vi "MainMeasure.vi"(0 "TestSeqClass.lvclass":refnum<class "TestSeqClass.lvclass">, 5 "error in (no error)":errorcluster, 7 "Handles_In":T3={"MHM_Handle in"=0, "axis in"={"keyHandle"=0, "nodeId"=1}}) -> (13 "Handles_Out":T2, 14 "TestSeqClass out":refnum<class "TestSeqClass.lvclass">, 15 "TestMeasureStep out":refnum<class "TestMeasureStep.lvclass">, 19 "error out":errorcluster)   [LabVIEW 2019]
uses:
  TestMeasureStep/TestMeasureStep.lvclass
  testSeq/TestSeqClass.lvclass
  testSeq/TestSeqClass.lvclass/TestSeqClass.ctl
  GUIHandler_Main/GUI_Handler_Main.lvclass/GUI_Handler_Main.ctl
  ProgramSettings/ProgramSettings.lvclass/ProgramSettings.ctl
  testSeq/Typedef/TestStatus.ctl
  DUT_Interface/lv_interface/enums/MHM_WriteVerifyEnum.ctl
  DUT_Interface/lv_interface/enums/MHM_ParamEnum.ctl
  02676b47-250f-4f2d-8756-12bf81697de7.vi
  ProgramSettings/ProgramSettings.lvclass
  GUIHandler_Main/GUI_Handler_Main.lvclass
  DUT_Interface/lv_interface/MHM_1SL_interface.lvlib
  InstrumentsInterfaces/Motordriver/maxon EPOS/Examples/maxonEPOS.lvlib
  <instrlib>/Scancon ASIC/Scancon ASIC.lvlib
panel:
  in  "communication settings in":T1={"deviceName"="EPOS4", "protocolStackName"="MAXON SERIAL V2", "interfaceName"="USB", "portName"="USB0", "baudrate"=1000000, "timeout"=100}
  in  "UseCurrentTestPointer":bool=TRUE
  out "index":i32
  in  "Combo Box":string(combo)
  in  "nodeId":u32=1
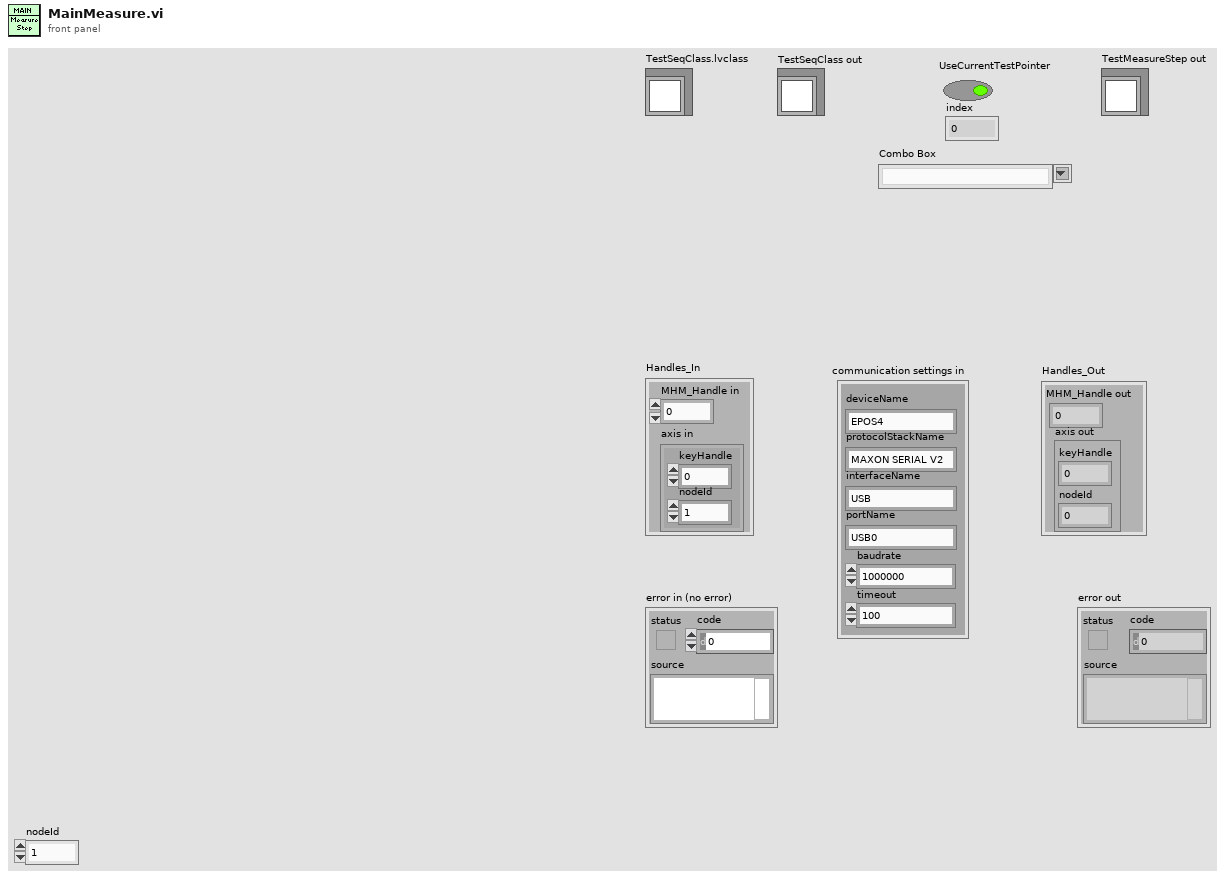
[diagram p1: front panel]
types:
  T1 = cluster{"deviceName":string, "protocolStackName":string, "interfaceName":string, "portName":string, "baudrate":u32, "timeout":u32}
  T2 = cluster{"MHM_Handle out":u32, "axis out":cluster{"keyHandle":u32, "nodeId":u16}}
  T3 = cluster{"MHM_Handle in":u32, "axis in":cluster{"keyHandle":u32, "nodeId":u16}}
  T4 = typedef "TestSeqType.ctl" = refnum<class "TestMeasureStep.lvclass">[]
  T5 = typedef "TestSeqClass.lvclass/TesstepType.ctl" = cluster{"TestName":string, "Meas":dbl, "Min ":dbl, "Max":dbl, "TestStatus":T6, "StringLimit":string, "StringMeas":string, "Unit":string}
  T6 = typedef "TestStatus.ctl" = enum16{"Not Executed", "Passed", "Failed", "Inconclusive", "Processing"}
  T7 = enum16{"MHM_NO_INTERFACE", "MHM_MB3U_SPI", "MHM_MB3U_BISS", "MHM_MB4U", "MHM_MB5U"}
  T8 = cluster{"profileAcceleration":u32, "profileDeceleration":u32}
  T9 = typedef "MHM_WriteVerifyEnum.ctl" = enum16{"MHM_SETONLY", "MHM_WRITE", "MHM_VERIFY"}
  T10 = typedef "MHM_ParamEnum.ctl" = enum16{"MHM_AVGFILT", "MHM_TLF", "MHM_DIR", "MHM_HYS", "MHM_RESO_MT", "MHM_RESO_ST", "MHM_CF_MTI", "MHM_SBL_MTI", "MHM_EBL_MTI", "MHM_GET_MTI", "MHM_CFG_IOP", "MHM_MT12", "MHM_RTX_MODE", "MHM_BIN_SSI", "MHM_EXT_SSI", "MHM_ENSSI", "MHM_VOSS", "MHM_VOSC", "MHM_CIBM", "MHM_ENF", "MHM_TEST", "MHM_GAINF", "MHM_GAINR", "MHM_GCC", "MHM_ENAC", "MHM_CRCS", "MHM_ENLC", "MHM_REGPROT", "MHM_INSPROT", "MHM_PRES_IO1", "MHM_DIR_IO2", "MHM_ENCMD3", "MHM_ENCMD2", "MHM_CRC_CFG", "MHM_OFFS_MT", "MHM_OFFS_ST", "MHM_CRC_OFFS", "MHM_PSET_MT", "MHM_PSET_ST", "MHM_CRC_PSET", "MHM_ERR_CFG", "MHM_ERR_OFFS", "MHM_ERR_POS", "MHM_ERR_EXT", "MHM_ERR_AMIN", "MHM_ERR_AMAX", "MHM_ERR_MTI", "MHM_ERR_MT", "MHM_GAIN", "MHM_EDSBANK", "MHM_PRO_ID", "MHM_DEV_ID0", "MHM_DEV_ID1", "MHM_DEV_ID2", "MHM_DEV_ID3", "MHM_DEV_ID4", "MHM_DEV_ID5", "MHM_MFG_ID0", "MHM_MFG_ID1", "MHM_HARMCAL", "MHM_DISBISS", "MHM_NTOA", "MHM_ENCMD01", "MHM_CHIP_REL"}
  T11 = cluster{"Konfigurations Filnavn":refnum<vi>, "Forsyningsspænding":refnum<vi>, "Kode":refnum<vi>, "Opløsning":refnum<vi>}
  T12 = typedef "ProgramSettings.lvclass/SettingParams.ctl" = cluster{"Serial Port for strømforsyning":refnum<visa-resource-name>, "Serial Port for SSI Interface":refnum<visa-resource-name>}
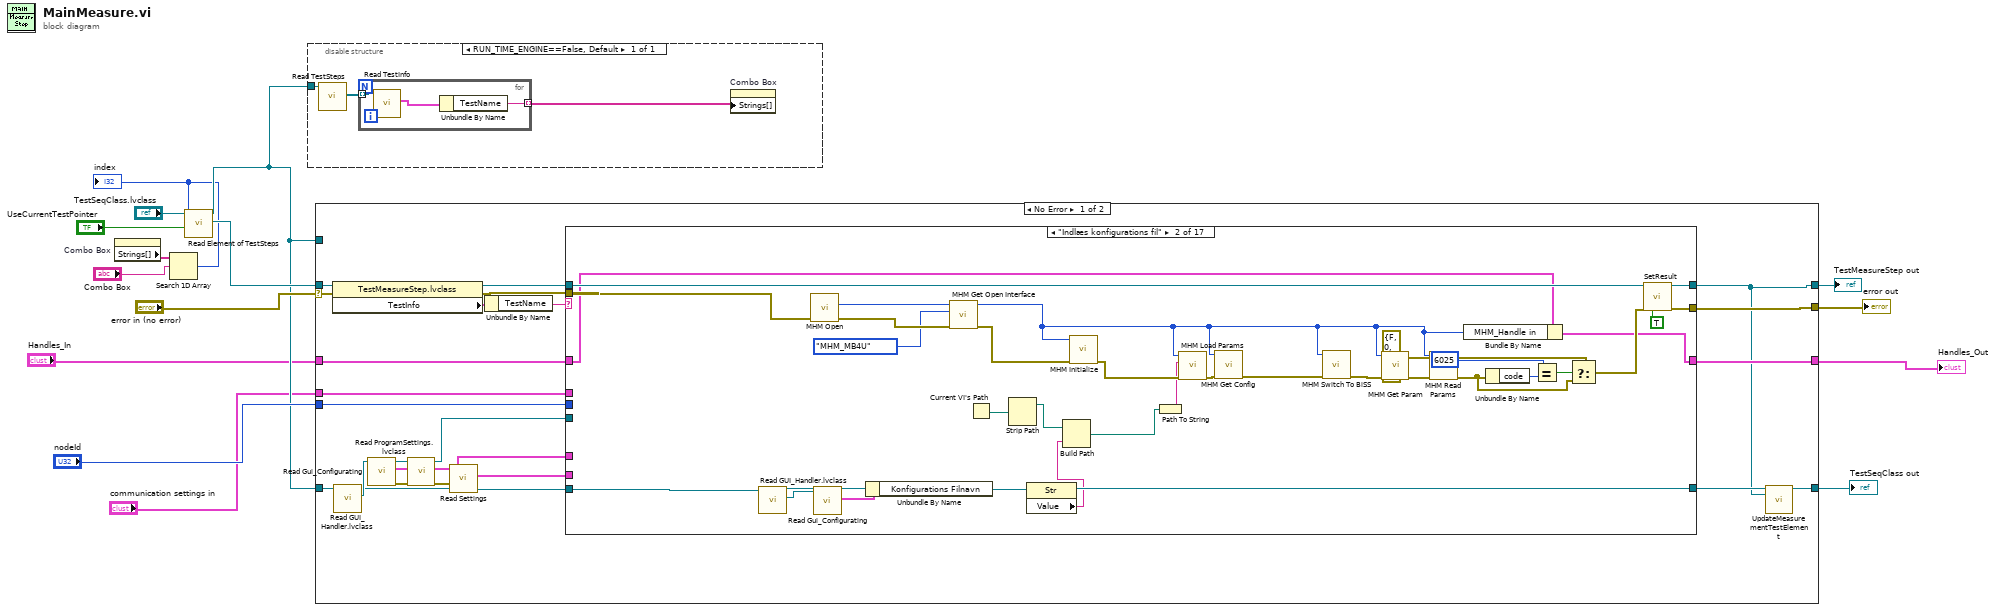
[diagram p0: block diagram]
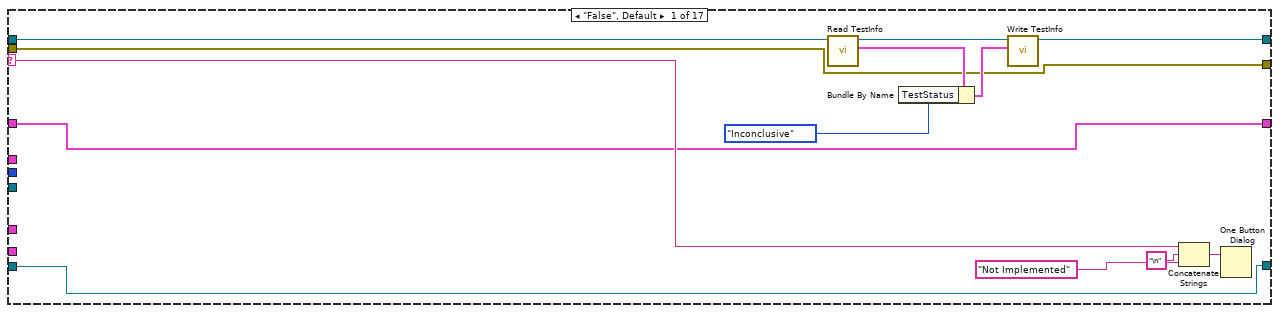
[diagram p2: hidden frame]
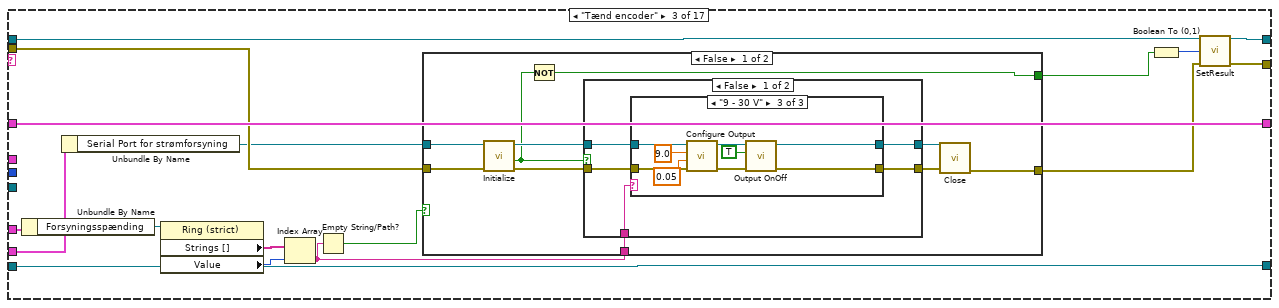
[diagram p3: hidden frame]
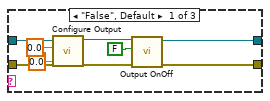
[diagram p4: hidden frame]
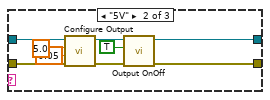
[diagram p5: hidden frame]
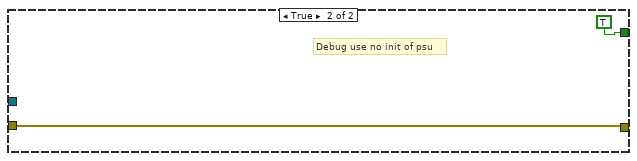
[diagram p7: hidden frame]
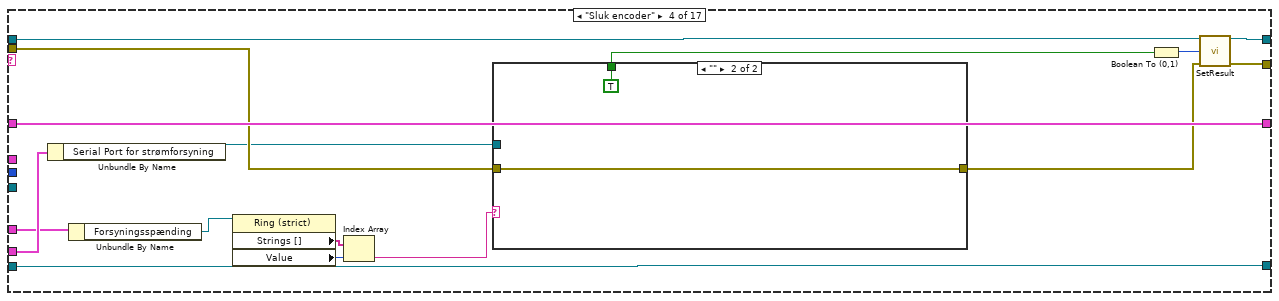
[diagram p8: hidden frame]
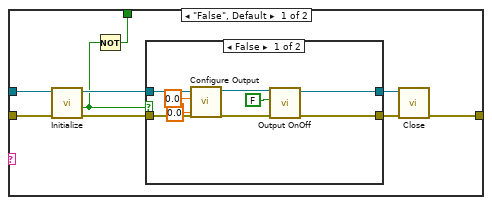
[diagram p9: hidden frame]
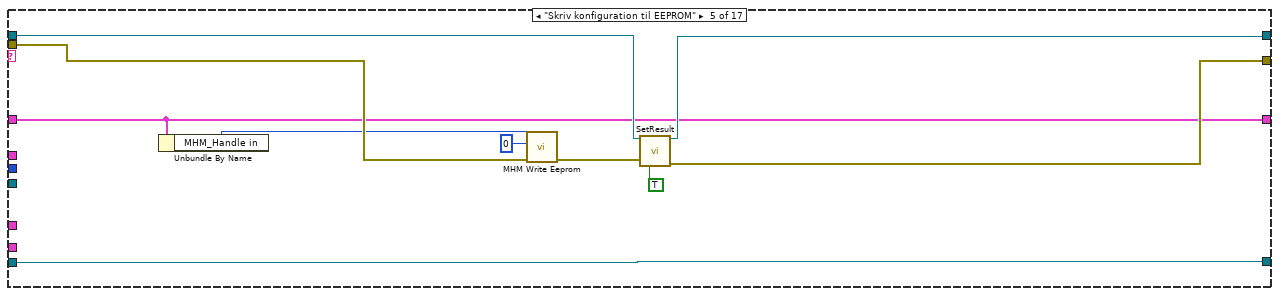
[diagram p11: hidden frame]
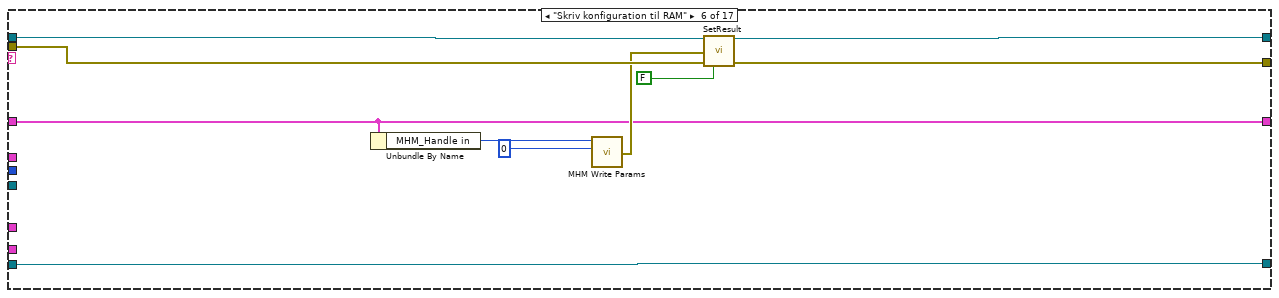
[diagram p12: hidden frame]
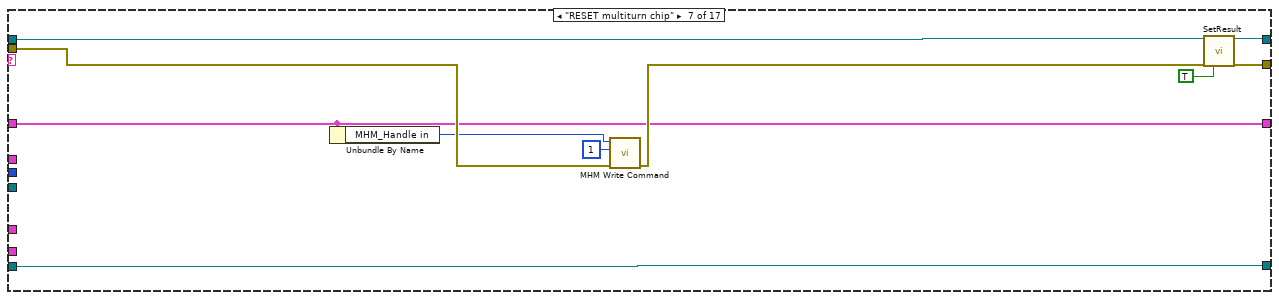
[diagram p13: hidden frame]
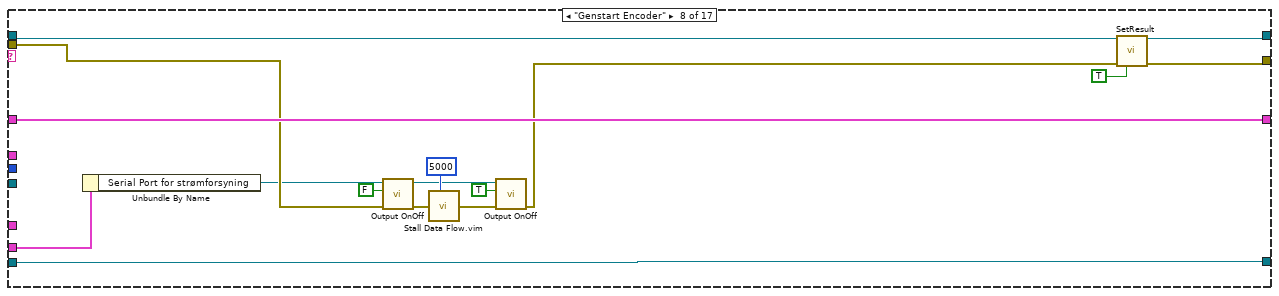
[diagram p14: hidden frame]
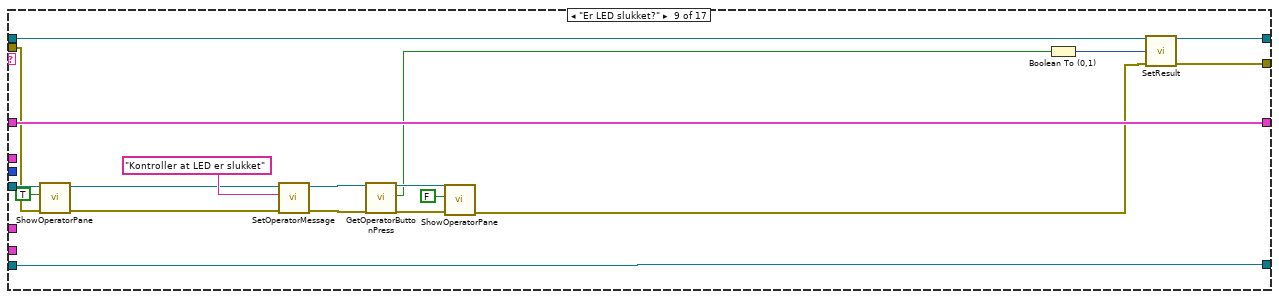
[diagram p15: hidden frame]
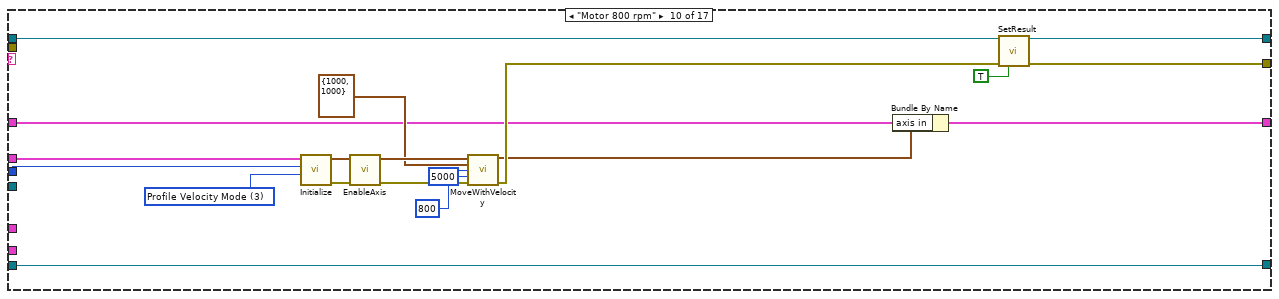
[diagram p16: hidden frame]
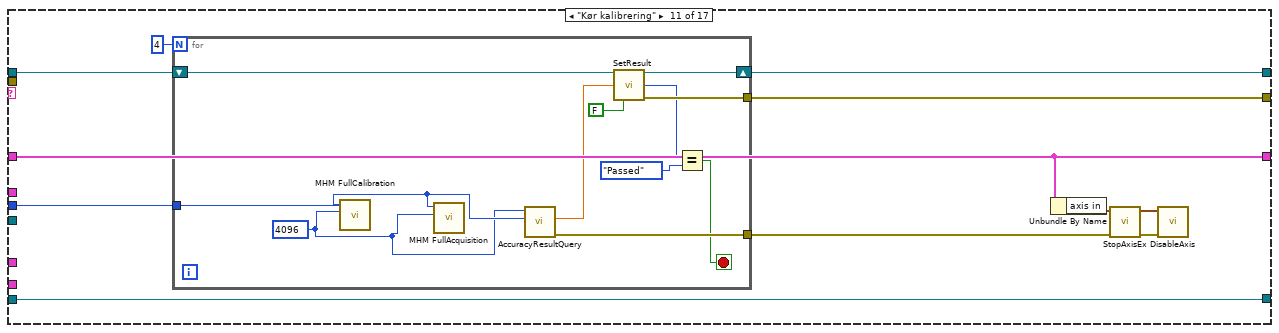
[diagram p17: hidden frame]
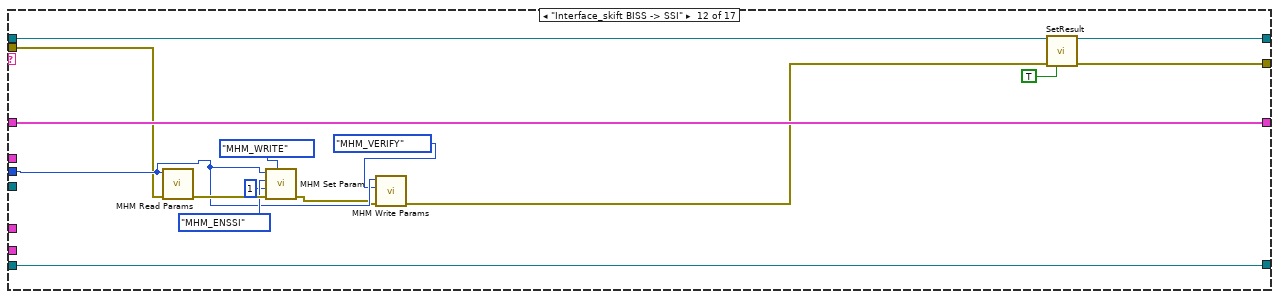
[diagram p18: hidden frame]
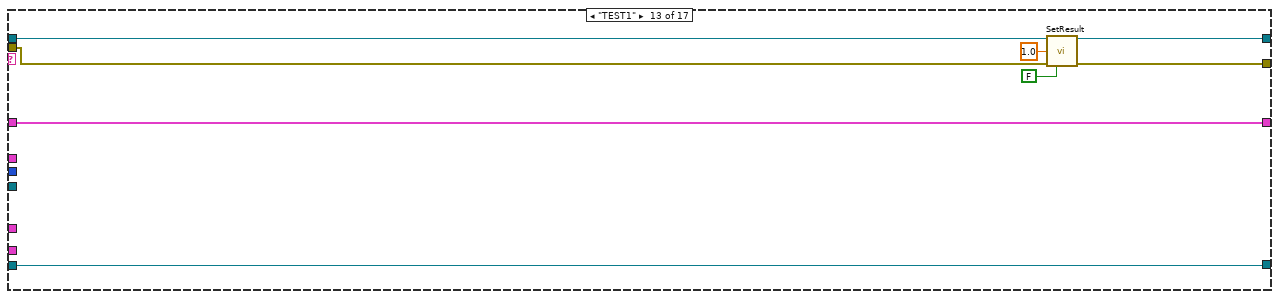
[diagram p19: hidden frame]
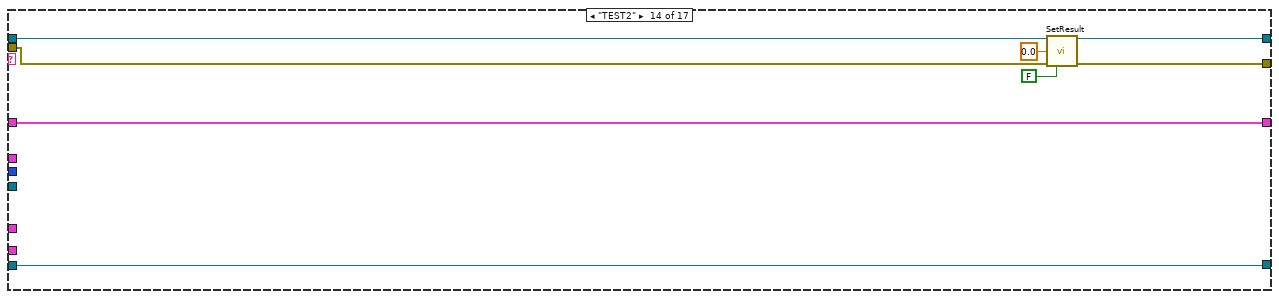
[diagram p20: hidden frame]
diagram:
  n1 = property on="Combo Box" class="CmbBox"() -> ("Strings[]"=w6:string[])  [unwired: 2 in, 2 out]
  n2 = Search 1D Array(1D array=w6, element="Combo Box") -> (index of element=w4:i32)  [unwired: 1 in]
  "index" <- w4
  n3 = call "Read Element of TestSteps.vi"("UseCurrentTestPointer"="UseCurrentTestPointer", "index"=w4, "TestSeqClass in"="TestSeqClass.lvclass") -> ("TestMeasureStep.lvclass"=w11:refnum<class "TestMeasureStep.lvclass">, "TestSeqClass out"=w8:refnum<class "TestSeqClass.lvclass">)  [unwired: 6 in, 1 out]
  n4 = disable-structure shown="RUN_TIME_ENGINE==False, Default" {
    disable-tunnel: w8 -> [w18]
    frame condition #0 (active) {
      n5 = call-dynamic "Read TestSteps.vi"("TestSeqClass in"=w18) -> ("TestSteps"=w17:T4)  [unwired: 8 in, 2 out]
      n6 = for {
        tunnel: w17 -> [w21] mode=indexing
        tunnel: [w19] -> w16 mode=indexing
        n7 = call-dynamic "Read TestInfo.vi"("TestMeasureStep in"=w21) -> ("TestInfo 2"=w20:T5)  [unwired: 8 in, 2 out]
        n8 = Unbundle By Name(w20) -> ("TestName"=w19:string)
      }
      n9 = property on="Combo Box" class="CmbBox"("Strings[]"=w16) -> ()  [unwired: 2 in, 2 out]
    }
  }
  n10 = case shown="No Error" "error in (no error)" {
    selector: "error in (no error)" -> [w38 w349]
    tunnel: [w36 w349] -> w14
    tunnel: [w33 w348] -> w13
    tunnel: w11 -> [w44 w348]
    tunnel: [w40 w347] -> w2
    tunnel: "Handles_In" -> [w39 w347]
    tunnel: w8 -> [w30 w346]
    tunnel: [w34 w346] -> w10
    tunnel: "nodeId" -> [w23 _]
    tunnel: w8 -> [_ _]
    tunnel: "communication settings in" -> [w22 _]
    frame No Error {
      n11 = property class="TestMeasureStep.lvclass"(reference=w44, error in=w38) -> (reference out=w42:refnum<class "TestMeasureStep.lvclass">, error out=w37:errorcluster, "TestInfo"=w43:T5)
      n12 = call-dynamic "Read GUI_Handler.lvclass.vi"("TestSeqClass in"=w30) -> ("GUI_Handler.lvclass"=w32:refnum<class "GUI_Handler_Main.lvclass">)  [unwired: 8 in, 2 out]
      n13 = call-dynamic "Read Gui_Configurating.vi"("GUI_Handler_Main in"=w32) -> ("error out"=w26:errorcluster, "Gui_Configurating"=w31:T11, "GUI_Handler_Main out"=w29:refnum<class "GUI_Handler_Main.lvclass">)  [unwired: 8 in]
      n14 = call "Read ProgramSettings.lvclass.vi"("error in (no error)"=w26, "GUI_Handler_Main in"=w29) -> ("error out"=w28:errorcluster, "ProgramSettings.lvclass"=w27:refnum<class "ProgramSettings.lvclass">, "GUI_Handler_Main out"=w24:refnum<class "GUI_Handler_Main.lvclass">)  [unwired: 7 in]
      n15 = call "Read Settings.vi"("error in (no error)"=w28, "ProgramSettings in"=w27) -> ("Settings"=w25:T12)  [unwired: 7 in, 2 out]
      n16 = Unbundle By Name(w43) -> ("TestName"=w41:string)
      n17 = case shown="\"Indlæs konfigurations fil\"" w41 {
        selector: w41 -> [w56 _ _ _ _ _ _ _ _ _ _ _ _ _ _ _ _]
        tunnel: w42 -> [w53 w90 w104 w165 w195 w204 w213 w221 w249 w260 w281 w304 w311 w319 w331 w336 w345]
        tunnel: [w48 w89 w103 w164 w192 w203 w212 w220 w248 w259 w280 w303 w310 w318 w331 w335 w345] -> w33
        tunnel: [w47 w60 w107 w168 w190 w200 w209 w233 w252 w254 w277 w308 w316 w324 w330 w341 w344] -> w40
        tunnel: w39 -> [w47 w59 w107 w168 w190 w200 w209 w233 w252 w255 w277 w308 w316 w324 w330 w341 w344]
        tunnel: w37 -> [w45 w88 w106 w167 w197 w207 w215 w231 w243 _ _ w295 w313 w321 w328 w332 w342]
        tunnel: w30 -> [w46 w87 w105 w166 w199 w208 w217 w232 w251 w271 w282 w307 w315 w323 w329 w340 w343]
        tunnel: [w46 w83 w105 w166 w199 w208 w217 w232 w251 w271 w282 w307 w315 w323 w329 w340 w343] -> w35
        tunnel: [w45 w82 w97 w159 w193 w207 w214 w219 w247 w258 w279 w306 w314 w322 w328 w334 w342] -> w36
        tunnel: w31 -> [_ _ w101 w157 _ _ _ _ _ _ _ _ _ _ _ _ _]
        tunnel: w25 -> [_ _ w100 w162 _ _ _ w230 _ _ _ _ _ _ w326 _ _]
        tunnel: w24 -> [_ _ _ _ _ _ _ _ w246 _ _ _ _ _ _ _ _]
        tunnel: w23 -> [_ _ _ _ _ _ _ _ _ w266 w278 w298 _ _ _ w339 _]
        tunnel: w22 -> [_ _ _ _ _ _ _ _ _ w253 _ _ _ _ _ _ _]
        frame "False", Default {
          n18 = call-dynamic "Read TestInfo.vi"("TestMeasureStep in"=w53) -> ("TestInfo 2"=w52:T5, "TestMeasureStep out"=w49:refnum<class "TestMeasureStep.lvclass">)  [unwired: 8 in, 1 out]
          n19 = Bundle By Name(cluster=w52, "TestStatus"=TestStatus."Inconclusive") -> (w50:T5)
          n20 = call-dynamic "Write TestInfo.vi"("TestInfo 2"=w50, "TestMeasureStep in"=w49) -> ("TestMeasureStep out"=w48:refnum<class "TestMeasureStep.lvclass">)  [unwired: 8 in, 1 out]
          n21 = Concatenate Strings(w56, "\n" ("string"), "Not Implemented" ("string")) -> (w57:string)
          n22 = One Button Dialog(message=w57) -> ()  [unwired: 1 in, 1 out]
        }
        frame "Indlæs konfigurations fil" {
          n23 = call-dynamic "Read GUI_Handler.lvclass.vi"("TestSeqClass in"=w87) -> ("GUI_Handler.lvclass"=w86:refnum<class "GUI_Handler_Main.lvclass">, "TestSeqClass out"=w83:refnum<class "TestSeqClass.lvclass">)  [unwired: 8 in, 1 out]
          n24 = call "MHM Open.vi"("error in (no error)"=w88) -> ("error out"=w65:errorcluster, "pulMHMHandle"=w62:u32)  [unwired: 8 in, 1 out]
          n25 = call-dynamic "Read Gui_Configurating.vi"("GUI_Handler_Main in"=w86) -> ("Gui_Configurating"=w85:T11)  [unwired: 8 in, 2 out]
          n26 = Unbundle By Name(w85) -> ("Konfigurations Filnavn"=w84:refnum<vi>)
          n27 = call "MHM Get Open Interface.vi"("error in (no error)"=w65, "ulInterface"=T7."MHM_MB4U" ("MHM_InterfaceEnum"), "ulMHMHandle"=w62) -> ("error out"=w64:errorcluster, "ulMHMHandle out"=w58:u32)  [unwired: 7 in]
          n28 = Current VI's Path() -> (path=w67:path)
          n29 = Strip Path(path=w67) -> (stripped path=w66:path)  [unwired: 1 out]
          n30 = property class="Str"(reference=w84) -> ("Value"=w69:string)  [unwired: 1 in, 2 out]
          n31 = Build Path(base path=w66, name or relative path=w69) -> (appended path=w68:path)
          n32 = call "MHM Initialize.vi"("error in (no error)"=w64, "ulMHMHandle"=w58) -> ("error out"=w81:errorcluster)  [unwired: 8 in, 1 out]
          n33 = Path To String(path=w68) -> (string=w70:string)
          n34 = call "MHM Load Params.vi"("error in (no error)"=w81, "pcFilename"=w70, "ulMHMHandle"=w58) -> ("error out"=w71:errorcluster)  [unwired: 7 in, 1 out]
          n35 = call "MHM Get Config.vi"("error in (no error)"=w71, "ulMHMHandle"=w58) -> ("error out"=w72:errorcluster)  [unwired: 7 in, 2 out]
          n36 = call "MHM Switch To BiSS.vi"("error in (no error)"=w72, "ulMHMHandle"=w58) -> ("error out"=w73:errorcluster)  [unwired: 7 in, 2 out]
          n37 = call "MHM Get Param.vi"("error in (no error)"=w73, "ulMHMHandle"=w58) -> ("error out"=w74:errorcluster)  [unwired: 7 in, 2 out]
          n38 = call "MHM Read Params.vi"("error in (no error)"=w74, "ulMHMHandle"=w58) -> ("error out"=w75:errorcluster)  [unwired: 8 in, 1 out]
          n39 = Bundle By Name(cluster=w59, "MHM_Handle in"=w58) -> (w60:T3)
          n40 = Unbundle By Name(w75) -> ("code"=w80:i32)
          n41 = Equal?(x=6025, y=w80) -> (x = y?=w78:bool)
          n42 = Select(t=errorcluster {"status"=FALSE, "code"=0, "source"=""}, s=w78, f=w75) -> (s? t:f=w76:errorcluster)
          n43 = call "SetResult.vi"("TestMeasureStep in"=w90, "error in (no error)"=w76, "Use Error As result"=TRUE) -> ("TestMeasureStep out"=w89:refnum<class "TestMeasureStep.lvclass">, "error out"=w82:errorcluster)  [unwired: 10 in, 1 out]
        }
        frame "Tænd encoder" {
          n44 = Unbundle By Name(w101) -> ("Forsyningsspænding"=w96:refnum<vi>)
          n45 = Unbundle By Name(w100) -> ("Serial Port for strømforsyning"=w99:refnum<visa-resource-name>)
          n46 = property class="Ring (strict)"(reference=w96) -> ("Strings []"=w95:string[], "Value"=w94:u16)  [unwired: 1 in, 2 out]
          n47 = Index Array(array=w95, index=w94) -> (element=w93:string)
          n48 = Empty String/Path?(string/path=w93) -> (empty?=w92:bool)
          n49 = case shown="False" w92 {
            tunnel: w106 -> [w117 w152]
            tunnel: w99 -> [w113 _]
            tunnel: [w112 w152] -> w98
            tunnel: w93 -> [w111 _]
            tunnel: [w108 TRUE ("Init failed")] -> w91
            frame False {
              n50 = call <instrlib>:"Initialize.vi"("error in (no error)"=w117, "VISA resource name"=w113) -> ("error out"=w110:errorcluster, "Init failed"=w109:bool, "VISA resource name out"=w116:refnum<visa-resource-name>)  [unwired: 6 in, 1 out]
              n51 = Not(x=w109) -> (.not. x?=w108:bool)
              n52 = case shown="False" w109 {
                tunnel: w116 -> [w122 w150]
                tunnel: w110 -> [w121 w149]
                tunnel: [w120 w150] -> w115
                tunnel: [w119 w149] -> w114
                tunnel: w111 -> [w118 _]
                frame False {
                  n53 = case shown="\"9 - 30 V\"" w118 {
                    tunnel: w122 -> [w126 w139 w148]
                    tunnel: w121 -> [w129 w133 w142]
                    tunnel: [w128 w136 w145] -> w120
                    tunnel: [w127 w132 w141] -> w119
                    frame "False", Default {
                      n54 = call <instrlib>:"Configure Output.vi"("Current Level (0.0 A)"=0.0, "Voltage Level (0.0 V)"=0.0, "VISA resource name"=w126) -> ("VISA resource name out"=w125:refnum<visa-resource-name>)  [unwired: 7 in, 1 out]
                      n55 = call <instrlib>:"Output OnOff.vi"("error in (no error)"=w129, "Output On/Off"=FALSE, "VISA resource name"=w125) -> ("error out"=w127:errorcluster, "VISA resource name out"=w128:refnum<visa-resource-name>)  [unwired: 7 in]
                    }
                    frame "5V" {
                      n56 = call <instrlib>:"Configure Output.vi"("error in (no error)"=w133, "Current Level (0.0 A)"=0.05, "Voltage Level (0.0 V)"=5.0, "VISA resource name"=w139) -> ("error out"=w135:errorcluster, "VISA resource name out"=w138:refnum<visa-resource-name>)  [unwired: 6 in]
                      n57 = call <instrlib>:"Output OnOff.vi"("error in (no error)"=w135, "Output On/Off"=TRUE, "VISA resource name"=w138) -> ("error out"=w132:errorcluster, "VISA resource name out"=w136:refnum<visa-resource-name>)  [unwired: 7 in]
                    }
                    frame "9 - 30 V" {
                      n58 = call <instrlib>:"Configure Output.vi"("error in (no error)"=w142, "Current Level (0.0 A)"=0.05, "Voltage Level (0.0 V)"=9.0, "VISA resource name"=w148) -> ("error out"=w144:errorcluster, "VISA resource name out"=w147:refnum<visa-resource-name>)  [unwired: 6 in]
                      n59 = call <instrlib>:"Output OnOff.vi"("error in (no error)"=w144, "Output On/Off"=TRUE, "VISA resource name"=w147) -> ("error out"=w141:errorcluster, "VISA resource name out"=w145:refnum<visa-resource-name>)  [unwired: 7 in]
                    }
                  }
                }
                frame True {
                }
              }
              n60 = call <instrlib>:"Close.vi"("error in (no error)"=w114, "VISA resource name"=w115) -> ("error out"=w112:errorcluster)  [unwired: 9 in]
            }
            frame True {
              # "Debug use no init of psu"
            }
          }
          n61 = Boolean To (0,1)(Boolean=w91) -> (0, 1=w102:i16)
          n62 = call "SetResult.vi"("TestMeasureStep in"=w104, "Meas"=w102, "error in (no error)"=w98) -> ("TestMeasureStep out"=w103:refnum<class "TestMeasureStep.lvclass">, "error out"=w97:errorcluster)  [unwired: 10 in, 1 out]
        }
        frame "Sluk encoder" {
          n63 = Unbundle By Name(w162) -> ("Serial Port for strømforsyning"=w161:refnum<visa-resource-name>)
          n64 = Unbundle By Name(w157) -> ("Forsyningsspænding"=w156:refnum<vi>)
          n65 = property class="Ring (strict)"(reference=w156) -> ("Strings []"=w154:string[], "Value"=w155:u16)  [unwired: 1 in, 2 out]
          n66 = Index Array(array=w154, index=w155) -> (element=w153:string)
          n67 = case shown="\"\"" w153 {
            tunnel: w167 -> [w177 w188]
            tunnel: w161 -> [w171 _]
            tunnel: [w170 w188] -> w160
            tunnel: [w169 TRUE] -> w158
            frame "False", Default {
              n68 = call <instrlib>:"Initialize.vi"("error in (no error)"=w177, "VISA resource name"=w171) -> ("error out"=w175:errorcluster, "Init failed"=w172:bool, "VISA resource name out"=w176:refnum<visa-resource-name>)  [unwired: 6 in, 1 out]
              n69 = Not(x=w172) -> (.not. x?=w169:bool)
              n70 = case shown="False" w172 {
                tunnel: w176 -> [w185 w187]
                tunnel: w175 -> [w184 w186]
                tunnel: [w183 w187] -> w174
                tunnel: [w182 w186] -> w173
                frame False {
                  n71 = call <instrlib>:"Configure Output.vi"("Current Level (0.0 A)"=0.0, "Voltage Level (0.0 V)"=0.0, "VISA resource name"=w185) -> ("VISA resource name out"=w180:refnum<visa-resource-name>)  [unwired: 7 in, 1 out]
                  n72 = call <instrlib>:"Output OnOff.vi"("error in (no error)"=w184, "Output On/Off"=FALSE, "VISA resource name"=w180) -> ("error out"=w182:errorcluster, "VISA resource name out"=w183:refnum<visa-resource-name>)  [unwired: 7 in]
                }
                frame True {
                }
              }
              n73 = call <instrlib>:"Close.vi"("error in (no error)"=w173, "VISA resource name"=w174) -> ("error out"=w170:errorcluster)  [unwired: 9 in]
            }
            frame "" {
            }
          }
          n74 = Boolean To (0,1)(Boolean=w158) -> (0, 1=w163:i16)
          n75 = call "SetResult.vi"("TestMeasureStep in"=w165, "Meas"=w163, "error in (no error)"=w160) -> ("TestMeasureStep out"=w164:refnum<class "TestMeasureStep.lvclass">, "error out"=w159:errorcluster)  [unwired: 10 in, 1 out]
        }
        frame "Skriv konfiguration til EEPROM" {
          n76 = Unbundle By Name(w190) -> ("MHM_Handle in"=w191:u32)
          n77 = call "MHM Write Eeprom.vi"("error in (no error)"=w197, "ulEepromArea"=u32 0, "ulMHMHandle"=w191) -> ("error out"=w196:errorcluster)  [unwired: 7 in, 1 out]
          n78 = call "SetResult.vi"("TestMeasureStep in"=w195, "error in (no error)"=w196, "Use Error As result"=TRUE) -> ("TestMeasureStep out"=w192:refnum<class "TestMeasureStep.lvclass">, "error out"=w193:errorcluster)  [unwired: 10 in, 1 out]
        }
        frame "Skriv konfiguration til RAM" {
          n79 = Unbundle By Name(w200) -> ("MHM_Handle in"=w201:u32)
          n80 = call "MHM Write Params.vi"("ulVerify"=u32 0, "ulMHMHandle"=w201) -> ("error out"=w205:errorcluster)  [unwired: 7 in, 2 out]
          n81 = call "SetResult.vi"("TestMeasureStep in"=w204, "error in (no error)"=w205, "Use Error As result"=FALSE) -> ("TestMeasureStep out"=w203:refnum<class "TestMeasureStep.lvclass">)  [unwired: 10 in, 2 out]
        }
        frame "RESET multiturn chip" {
          n82 = Unbundle By Name(w209) -> ("MHM_Handle in"=w210:u32)
          n83 = call "MHM Write Command.vi"("error in (no error)"=w215, "ulCommand"=u32 1, "ulMHMHandle"=w210) -> ("error out"=w214:errorcluster)  [unwired: 7 in, 1 out]
          n84 = call "SetResult.vi"("TestMeasureStep in"=w213, "Use Error As result"=TRUE) -> ("TestMeasureStep out"=w212:refnum<class "TestMeasureStep.lvclass">)  [unwired: 11 in, 2 out]
        }
        frame "Genstart Encoder" {
          n85 = Unbundle By Name(w230) -> ("Serial Port for strømforsyning"=w229:refnum<visa-resource-name>)
          n86 = call <instrlib>:"Output OnOff.vi"("error in (no error)"=w231, "Output On/Off"=FALSE, "VISA resource name"=w229) -> ("error out"=w227:errorcluster, "VISA resource name out"=w224:refnum<visa-resource-name>)  [unwired: 7 in]
          n87 = call "Stall Data Flow.vim"("value in"=w227, "milliseconds to wait"=u32 5000) -> ("value out"=w225:errorcluster)  [unwired: 1 out]
          n88 = call <instrlib>:"Output OnOff.vi"("error in (no error)"=w225, "Output On/Off"=TRUE, "VISA resource name"=w224) -> ("error out"=w222:errorcluster)  [unwired: 7 in, 1 out]
          n89 = call "SetResult.vi"("TestMeasureStep in"=w221, "error in (no error)"=w222, "Use Error As result"=TRUE) -> ("TestMeasureStep out"=w220:refnum<class "TestMeasureStep.lvclass">, "error out"=w219:errorcluster)  [unwired: 10 in, 1 out]
        }
        frame "Er LED slukket?" {
          n90 = call-dynamic "ShowOperatorPane.vi"("error in (no error)"=w243, "Visible"=TRUE, "GUI_Handler_Main in"=w246) -> ("error out"=w244:errorcluster, "GUI_Handler_Main out"=w245:refnum<class "GUI_Handler_Main.lvclass">)  [unwired: 7 in]
          n91 = call-dynamic "SetOperatorMessage.vi"("error in (no error)"=w244, "Value"="Kontroller at LED er slukket", "GUI_Handler_Main in"=w245) -> ("error out"=w241:errorcluster, "GUI_Handler_Main out"=w240:refnum<class "GUI_Handler_Main.lvclass">)  [unwired: 7 in]
          n92 = call-dynamic "GetOperatorButtonPress.vi"("GUI_Handler_Main in"=w240, "error in (no error)"=w241) -> ("GUI_Handler_Main out"=w237:refnum<class "GUI_Handler_Main.lvclass">, "Operator_Aceept"=w235:bool, "error out"=w238:errorcluster)  [unwired: 13 in, 2 out]
          n93 = call-dynamic "ShowOperatorPane.vi"("error in (no error)"=w238, "Visible"=FALSE, "GUI_Handler_Main in"=w237) -> ("error out"=w234:errorcluster)  [unwired: 7 in, 1 out]
          n94 = Boolean To (0,1)(Boolean=w235) -> (0, 1=w239:i16)
          n95 = call "SetResult.vi"("TestMeasureStep in"=w249, "Meas"=w239, "error in (no error)"=w234) -> ("TestMeasureStep out"=w248:refnum<class "TestMeasureStep.lvclass">, "error out"=w247:errorcluster)  [unwired: 10 in, 1 out]
        }
        frame "Motor 800 rpm" {
          w264 = i8 3 items=["Profile Position Mode"=1, "Profile Velocity Mode"=3, "Homing Mode"=6, "Interpolated Position Mode"=7, "Position Mode"=-1, "Velocity Mode"=-2, "Current Mode"=-3, "Master Encoder Mode"=-5, "Step Direction Mode"=-6] ("modes of operations")
          n96 = call <instrlib>:"Initialize.vi"("modes of operations"=w264, "nodeId"=w266, "communication settings in"=w253) -> ("error out"=w267:errorcluster, "axis out"=w269:cluster{"keyHandle":u32, "nodeId":u16})  [unwired: 7 in]
          n97 = call "EnableAxis.vi"("error in (no error)"=w267, "axis in"=w269) -> ("error out"=w268:errorcluster, "axis out"=w270:cluster{"keyHandle":u32, "nodeId":u16})  [unwired: 4 in]
          n98 = call "MoveWithVelocity.vi"("axis in"=w270, "velocity profile"=T8 {"profileAcceleration"=1000, "profileDeceleration"=1000}, "targetVelocity"=800, "timeout"=u32 5000, "error in (no error)"=w268) -> ("axis out"=w256:cluster{"keyHandle":u32, "nodeId":u16}, "error out"=w261:errorcluster)  [unwired: 9 in]
          n99 = Bundle By Name(cluster=w255, "axis in"=w256) -> (w254:T3)
          n100 = call "SetResult.vi"("TestMeasureStep in"=w260, "error in (no error)"=w261, "Use Error As result"=TRUE) -> ("TestMeasureStep out"=w259:refnum<class "TestMeasureStep.lvclass">, "error out"=w258:errorcluster)  [unwired: 10 in, 1 out]
        }
        frame "Kør kalibrering" {
          n101 = for {
            N: 4 -> [_]
            tunnel: [w291] -> w279
            tunnel: w278 -> [w289]
            tunnel: [w286] -> w276
            shift-right: [w292] -> w280
            shift-left: w281 -> [w293]
            stop <- w283 stop-if-true
            w288 = u32 4096 ("ulCycles")
            n102 = call "MHM FullCalibration.vi"("ulCycles"=w288, "ulMHMHandle"=w289) -> ()  [unwired: 8 in, 2 out]
            n103 = call "MHM FullAcquisition.vi"("ulCycles"=w288, "ulMHMHandle"=w289) -> ()  [unwired: 8 in, 2 out]
            n104 = call "AccuracyResultQuery.vi"("pulMHMHandle"=w289, "pulNumberOfBytes"=w288) -> ("error out"=w286:errorcluster, "Error Range"=w287:dbl)  [unwired: 5 in, 3 out]
            n105 = call "SetResult.vi"("TestMeasureStep in"=w293, "Meas"=w287, "Use Error As result"=FALSE) -> ("TestMeasureStep out"=w292:refnum<class "TestMeasureStep.lvclass">, "TestStatus"=w284:T6, "error out"=w291:errorcluster)  [unwired: 10 in]
            n106 = Equal?(x=w284, y=TestStatus."Passed" ("TestStatus")) -> (x = y?=w283:bool)
          }
          n107 = Unbundle By Name(w277) -> ("axis in"=w273:cluster{"keyHandle":u32, "nodeId":u16})
          n108 = call "StopAxisEx.vi"("error in (no error)"=w276, "axis in"=w273) -> ("error out"=w274:errorcluster, "axis out"=w272:cluster{"keyHandle":u32, "nodeId":u16})  [unwired: 4 in]
          n109 = call "DisableAxis.vi"("error in (no error)"=w274, "axis in"=w272) -> ()  [unwired: 4 in, 2 out]
        }
        frame "Interface_skift BISS -> SSI" {
          n110 = call "MHM Read Params.vi"("error in (no error)"=w295, "ulMHMHandle"=w298) -> ("error out"=w302:errorcluster)  [unwired: 8 in, 1 out]
          n111 = call "MHM Set Param.vi"("ulWriteVerify"=MHM_WriteVerifyEnum."MHM_WRITE" ("MHM_E2PRangeEnum"), "error in (no error)"=w302, "ulValue"=u32 1, "ulParam"=MHM_ParamEnum."MHM_ENSSI" ("MHM_ParamEnum"), "ulMHMHandle"=w298) -> ("error out"=w296:errorcluster)  [unwired: 5 in, 1 out]
          n112 = call "MHM Write Params.vi"("error in (no error)"=w296, "ulVerify"=MHM_WriteVerifyEnum."MHM_VERIFY" ("MHM_E2PRangeEnum"), "ulMHMHandle"=w298) -> ("error out"=w294:errorcluster)  [unwired: 6 in, 2 out]
          n113 = call "SetResult.vi"("TestMeasureStep in"=w304, "error in (no error)"=w294, "Use Error As result"=TRUE) -> ("TestMeasureStep out"=w303:refnum<class "TestMeasureStep.lvclass">, "error out"=w306:errorcluster)  [unwired: 10 in, 1 out]
        }
        frame "TEST1" {
          n114 = call "SetResult.vi"("TestMeasureStep in"=w311, "Meas"=1.0, "error in (no error)"=w313, "Use Error As result"=FALSE) -> ("TestMeasureStep out"=w310:refnum<class "TestMeasureStep.lvclass">, "error out"=w314:errorcluster)  [unwired: 9 in, 1 out]
        }
        frame "TEST2" {
          n115 = call "SetResult.vi"("TestMeasureStep in"=w319, "Meas"=0.0, "error in (no error)"=w321, "Use Error As result"=FALSE) -> ("TestMeasureStep out"=w318:refnum<class "TestMeasureStep.lvclass">, "error out"=w322:errorcluster)  [unwired: 9 in, 1 out]
        }
        frame "PING SSI interface" {
          n116 = Unbundle By Name(w326) -> ("Serial Port for SSI Interface"=w325:refnum<visa-resource-name>)
          n117 = call <instrlib>:"ASICtool open.vi"("VISA Refnum in"=w325) -> ("VISA Refnum out"=w327:refnum<visa-resource-name>)  [unwired: 9 in, 1 out]
          n118 = call <instrlib>:"ASICtool Ping.vi"("VISA Refnum in"=w327) -> ()  [unwired: 7 in, 4 out]
        }
        frame "Skriv Konfig til EEPROM" {
          n119 = call "MHM Write Eeprom.vi"("error in (no error)"=w332, "ulEepromArea"=u32 0, "ulMHMHandle"=w339) -> ("error out"=w333:errorcluster)  [unwired: 7 in, 1 out]
          n120 = call "SetResult.vi"("TestMeasureStep in"=w336, "error in (no error)"=w333, "Use Error As result"=TRUE) -> ("TestMeasureStep out"=w335:refnum<class "TestMeasureStep.lvclass">, "error out"=w334:errorcluster)  [unwired: 10 in, 1 out]
        }
        frame "Exit" {
        }
      }
      n121 = call "UpdateMeasurementTestElement.vi"("TestSeqClass in"=w35, "TestMeasureStep.lvclass"=w33) -> ("TestSeqClass out"=w34:refnum<class "TestSeqClass.lvclass">)  [unwired: 12 in, 1 out]
    }
    frame Error {
    }
  }
  "error out" <- w14
  "TestMeasureStep out" <- w13
  "TestSeqClass out" <- w10
  "Handles_Out" <- w2
